vi "Data_Save_ECO.vi"(9 "Data":T1) -> (2 "Eco":string[](array[string]))   [LabVIEW 2017]
uses:
  Ctrls/Data.ctl
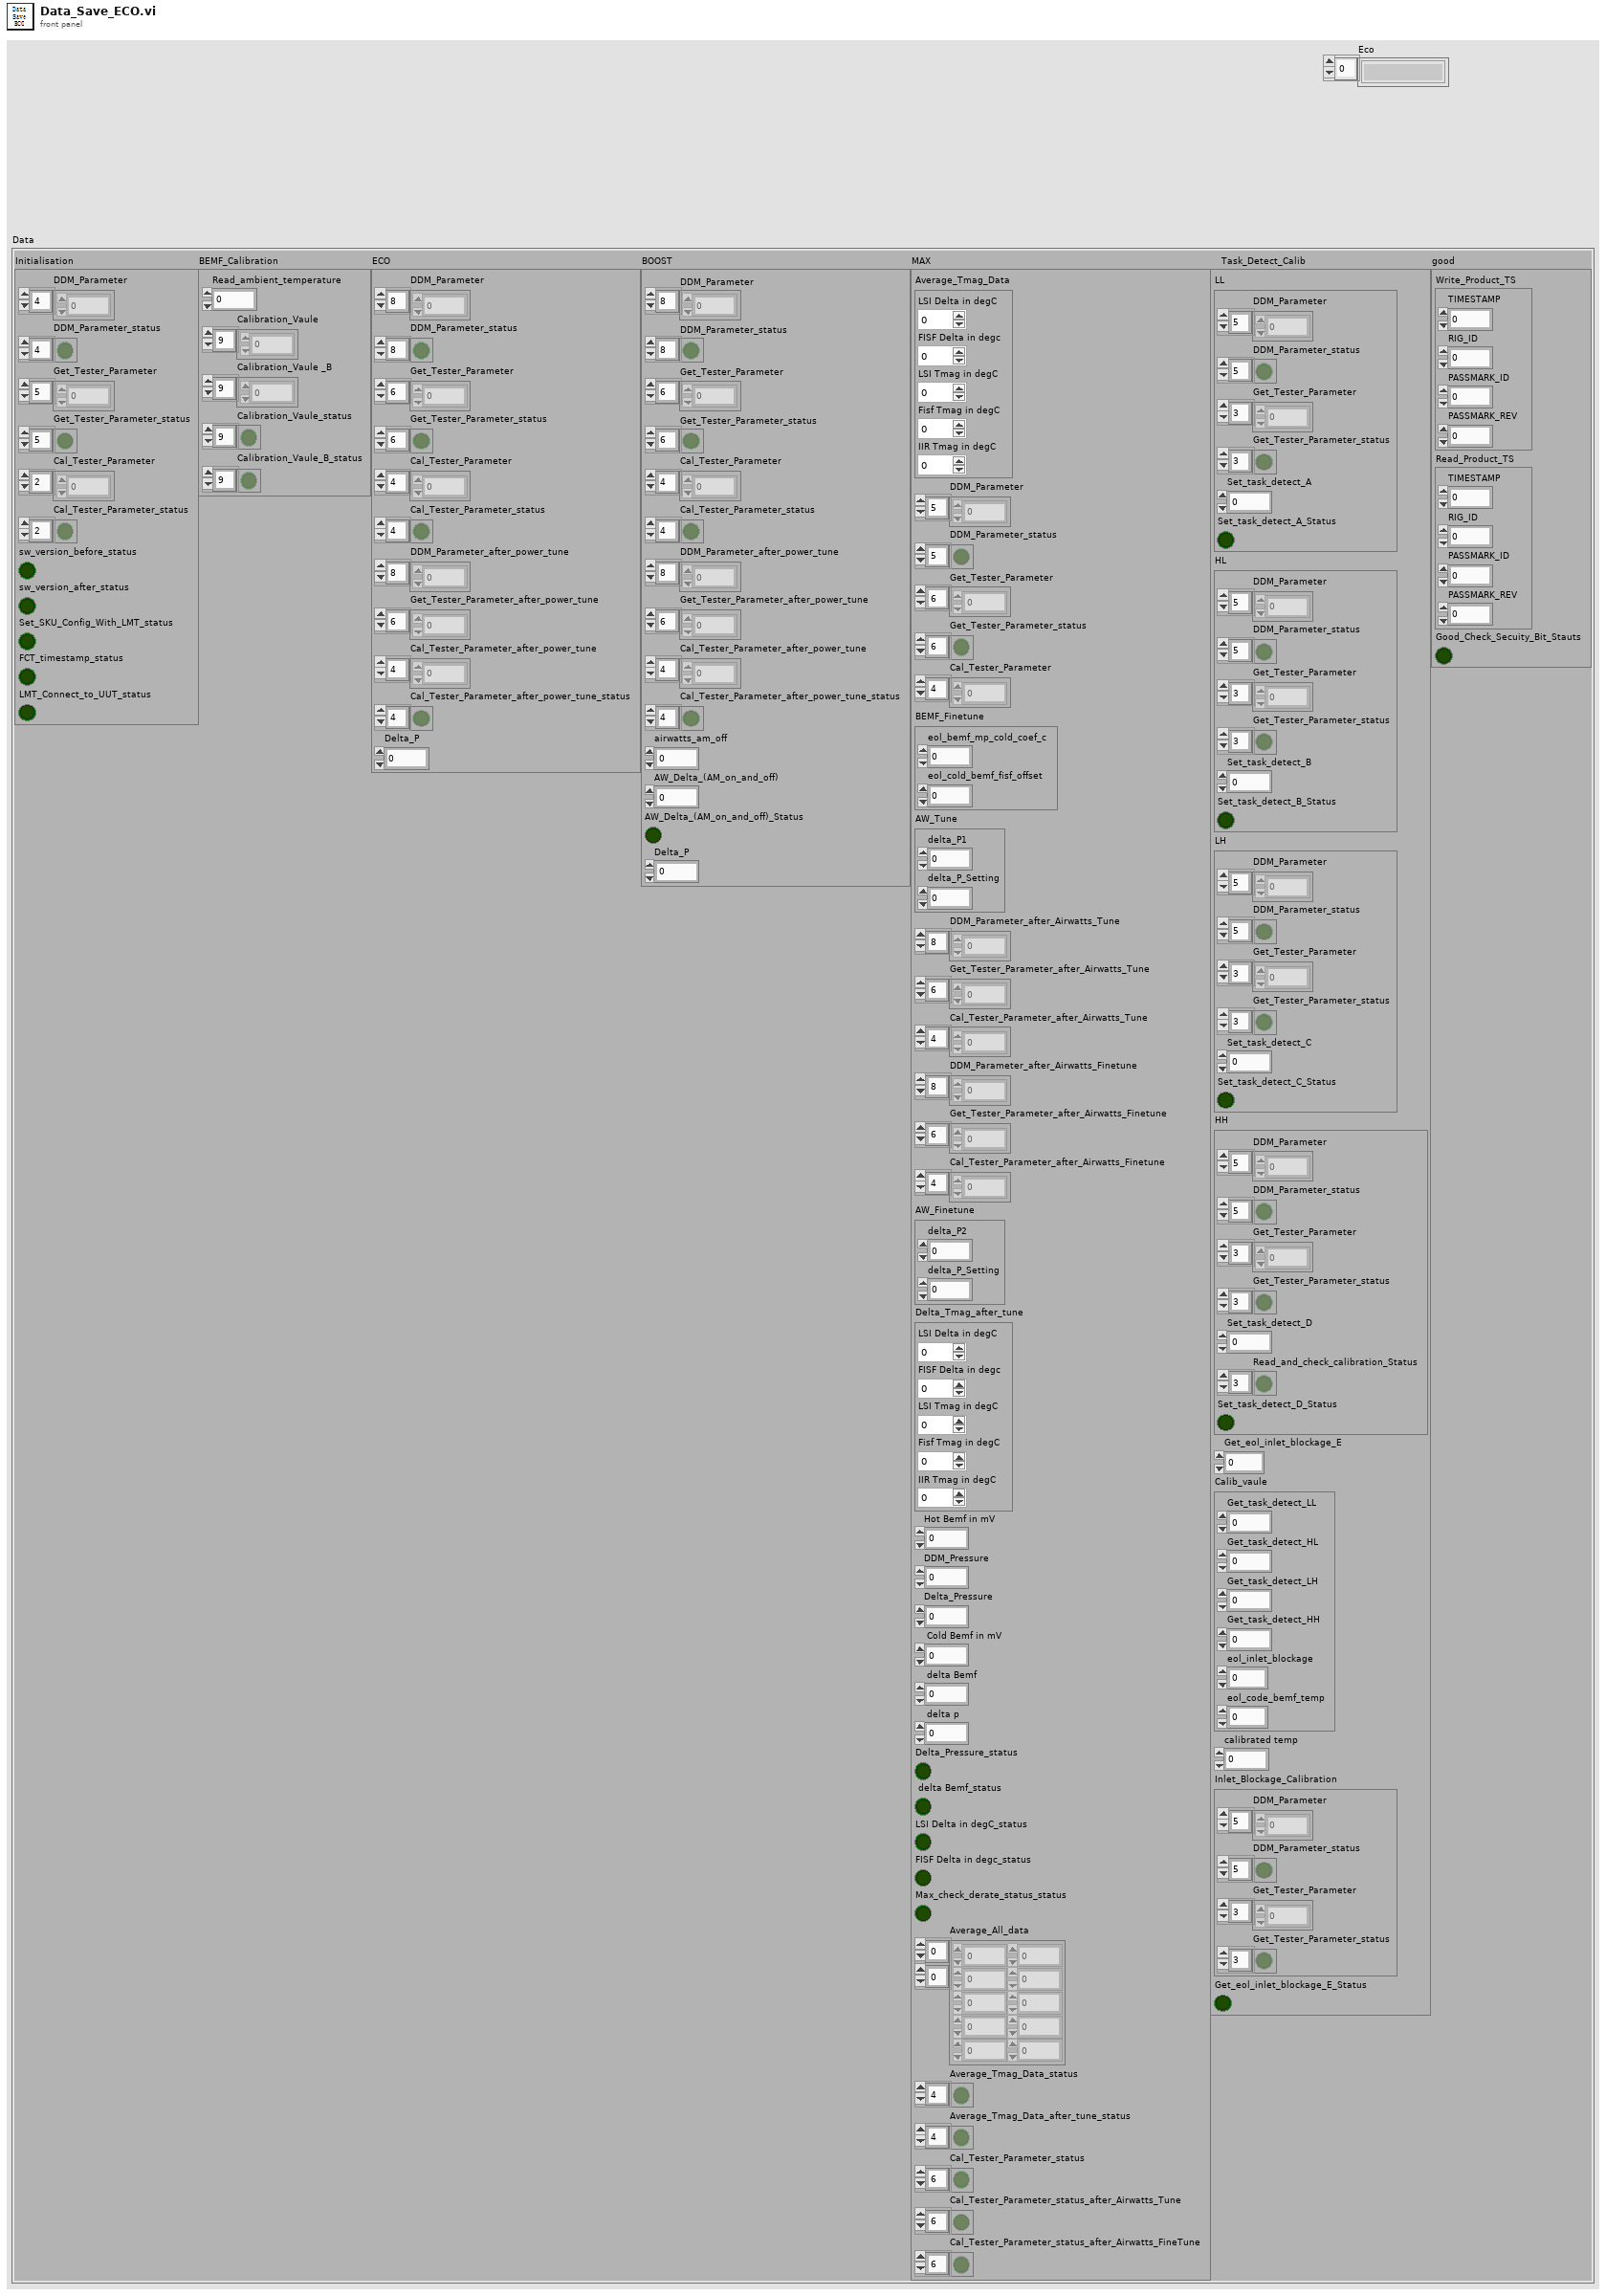
[diagram p1: front panel]
types:
  T1 = typedef "Data.ctl" = cluster{"Initialisation":cluster{"DDM_Parameter":dbl[], "DDM_Parameter_status":bool[], "Get_Tester_Parameter":dbl[], "Get_Tester_Parameter_status":bool[], "Cal_Tester_Parameter":dbl[], "Cal_Tester_Parameter_status":bool[], "sw_version_before_status":bool, "sw_version_after_status":bool, "Set_SKU_Config_With_LMT_status":bool, "FCT_timestamp_status":bool, "LMT_Connect_to_UUT_status":bool}, "BEMF_Calibration":cluster{"Read_ambient_temperature":dbl, "Calibration_Vaule":dbl[], "Calibration_Vaule _B":dbl[], "Calibration_Vaule_status":bool[], "Calibration_Vaule_B_status":bool[]}, "ECO":cluster{"DDM_Parameter":dbl[], "DDM_Parameter_status":bool[], "Get_Tester_Parameter":dbl[], "Get_Tester_Parameter_status":bool[], "Cal_Tester_Parameter":dbl[], "Cal_Tester_Parameter_status":bool[], "DDM_Parameter_after_power_tune":dbl[], "Get_Tester_Parameter_after_power_tune":dbl[], "Cal_Tester_Parameter_after_power_tune":dbl[], "Cal_Tester_Parameter_after_power_tune_status":bool[], "Delta_P":dbl}, "BOOST":cluster{"DDM_Parameter":dbl[], "DDM_Parameter_status":bool[], "Get_Tester_Parameter":dbl[], "Get_Tester_Parameter_status":bool[], "Cal_Tester_Parameter":dbl[], "Cal_Tester_Parameter_status":bool[], "DDM_Parameter_after_power_tune":dbl[], "Get_Tester_Parameter_after_power_tune":dbl[], "Cal_Tester_Parameter_after_power_tune":dbl[], "Cal_Tester_Parameter_after_power_tune_status":bool[], "airwatts_am_off":dbl, "AW_Delta_(AM_on_and_off)":dbl, "AW_Delta_(AM_on_and_off)_Status":bool, "Delta_P":dbl}, "MAX":cluster{"Average_Tmag_Data":cluster{"LSI Delta in degC":dbl, "FISF Delta in degc":dbl, "LSI Tmag in degC":dbl, "Fisf Tmag in degC":dbl, "IIR Tmag in degC":dbl}, "DDM_Parameter":dbl[], "DDM_Parameter_status":bool[], "Get_Tester_Parameter":dbl[], "Get_Tester_Parameter_status":bool[], "Cal_Tester_Parameter":dbl[], "BEMF_Finetune":cluster{"eol_bemf_mp_cold_coef_c":dbl, "eol_cold_bemf_fisf_offset":dbl}, "AW_Tune":cluster{"delta_P1":dbl, "delta_P_Setting":dbl}, "DDM_Parameter_after_Airwatts_Tune":dbl[], "Get_Tester_Parameter_after_Airwatts_Tune":dbl[], "Cal_Tester_Parameter_after_Airwatts_Tune":dbl[], "DDM_Parameter_after_Airwatts_Finetune":dbl[], "Get_Tester_Parameter_after_Airwatts_Finetune":dbl[], "Cal_Tester_Parameter_after_Airwatts_Finetune":dbl[], "AW_Finetune":cluster{"delta_P2":dbl, "delta_P_Setting":dbl}, "Delta_Tmag_after_tune":cluster{"LSI Delta in degC":dbl, "FISF Delta in degc":dbl, "LSI Tmag in degC":dbl, "Fisf Tmag in degC":dbl, "IIR Tmag in degC":dbl}, "Hot Bemf in mV":dbl, "DDM_Pressure":dbl, "Delta_Pressure":dbl, " Cold Bemf in mV":dbl, " delta Bemf":dbl, " delta p":dbl, "Delta_Pressure_status":bool, " delta Bemf_status":bool, "LSI Delta in degC_status":bool, "FISF Delta in degc_status":bool, "Max_check_derate_status_status":bool, "Average_All_data":dbl[][], "Average_Tmag_Data_status":bool[], "Average_Tmag_Data_after_tune_status":bool[], "Cal_Tester_Parameter_status":bool[], "Cal_Tester_Parameter_status_after_Airwatts_Tune":bool[], "Cal_Tester_Parameter_status_after_Airwatts_FineTune":bool[]}, "Task_Detect_Calib":cluster{"LL":cluster{"DDM_Parameter":dbl[], "DDM_Parameter_status":bool[], "Get_Tester_Parameter":dbl[], "Get_Tester_Parameter_status":bool[], "Set_task_detect_A":dbl, "Set_task_detect_A_Status":bool}, "HL":cluster{"DDM_Parameter":dbl[], "DDM_Parameter_status":bool[], "Get_Tester_Parameter":dbl[], "Get_Tester_Parameter_status":bool[], "Set_task_detect_B":dbl, "Set_task_detect_B_Status":bool}, "LH":cluster{"DDM_Parameter":dbl[], "DDM_Parameter_status":bool[], "Get_Tester_Parameter":dbl[], "Get_Tester_Parameter_status":bool[], "Set_task_detect_C":dbl, "Set_task_detect_C_Status":bool}, "HH":cluster{"DDM_Parameter":dbl[], "DDM_Parameter_status":bool[], "Get_Tester_Parameter":dbl[], "Get_Tester_Parameter_status":bool[], "Set_task_detect_D":dbl, "Read_and_check_calibration_Status":bool[], "Set_task_detect_D_Status":bool}, "Get_eol_inlet_blockage_E":dbl, "Calib_vaule":cluster{"Get_task_detect_LL":dbl, "Get_task_detect_HL":dbl, "Get_task_detect_LH":dbl, "Get_task_detect_HH":dbl, "eol_inlet_blockage":dbl, "eol_code_bemf_temp":dbl}, "calibrated temp":dbl, "Inlet_Blockage_Calibration":cluster{"DDM_Parameter":dbl[], "DDM_Parameter_status":bool[], "Get_Tester_Parameter":dbl[], "Get_Tester_Parameter_status":bool[]}, "Get_eol_inlet_blockage_E_Status":bool}, "good":cluster{"Write_Product_TS":cluster{"TIMESTAMP":i64, "RIG_ID":i64, "PASSMARK_ID":i64, "PASSMARK_REV":i64}, "Read_Product_TS":cluster{"TIMESTAMP":i64, "RIG_ID":i64, "PASSMARK_ID":i64, "PASSMARK_REV":i64}, "Good_Check_Secuity_Bit_Stauts":bool}}
  T2 = typedef "HD Config.ctl" = cluster{" PC":cluster{"PC Address":u8[], "PC Port":i32}, "FCO":cluster{"COM":refnum<visa-resource-name>, "Baudrate":u32}, "DC Power ":cluster{"COM":refnum<visa-resource-name>, "Baudrate":u32}, "PW3336":cluster{"COM":refnum<visa-resource-name>, "Baudrate":u32}, "Lefoo":cluster{"COM":refnum<visa-resource-name>, "Baudrate":u32}, "AI Model":cluster{"COM":refnum<visa-resource-name>, "Baudrate":u32}, "DIPC":cluster{"COM":refnum<visa-resource-name>}, "Daemon":cluster{"IP Address":string, "Port":u16, "Retry":u16}, "Motor":cluster{"COM":refnum<visa-resource-name>, "Baudrate":u32}, "G1":bool, "Fail_resume_mode":bool, "Skip DDM Speed&Pressure Passmark":bool}
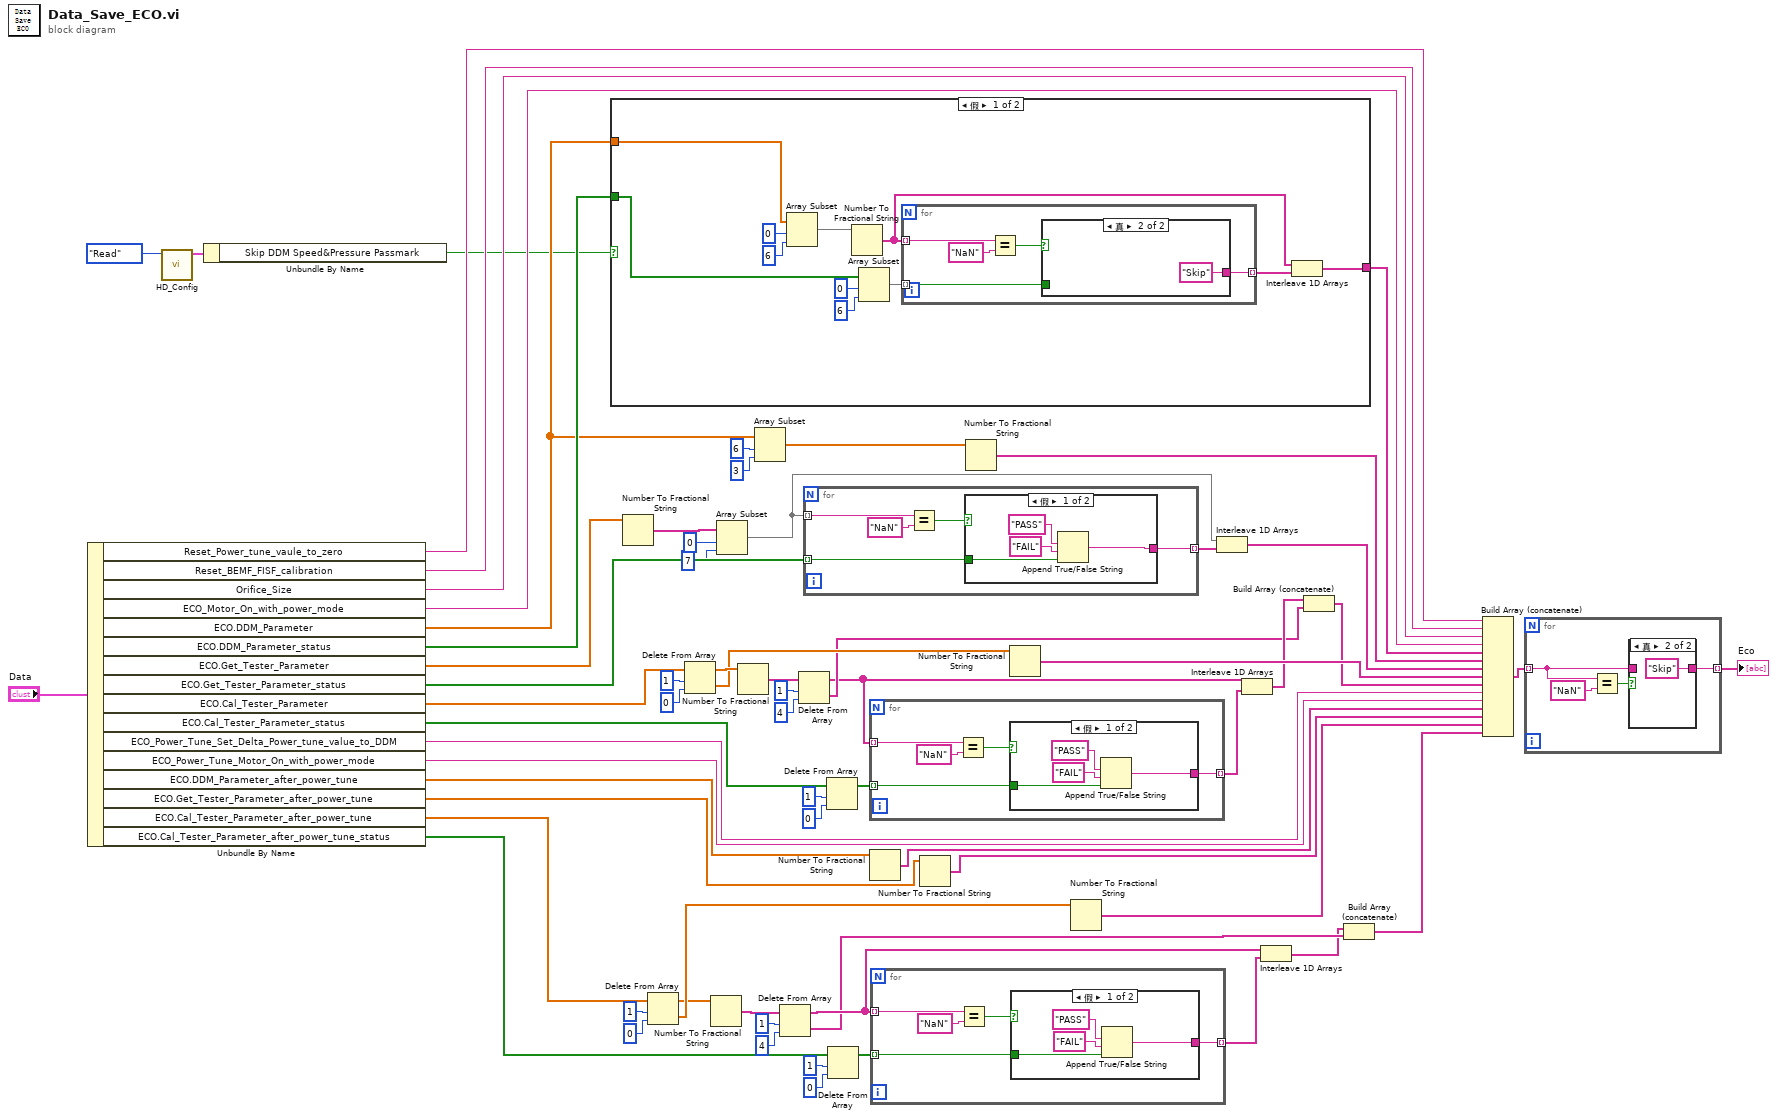
[diagram p0: block diagram]
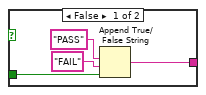
[diagram p2: hidden frame]
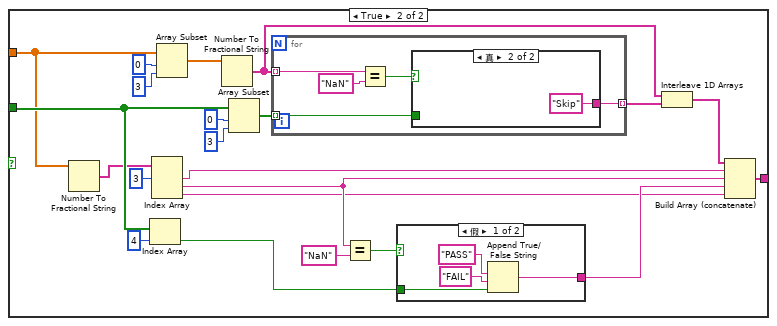
[diagram p3: hidden frame]
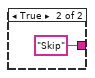
[diagram p4: hidden frame]
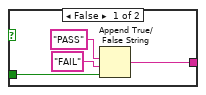
[diagram p5: hidden frame]
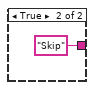
[diagram p7: hidden frame]
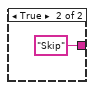
[diagram p8: hidden frame]
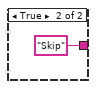
[diagram p9: hidden frame]
diagram:
  n1 = Unbundle By Name("Data") -> ("Reset_Power_tune_vaule_to_zero"=w28:string, "Reset_BEMF_FISF_calibration"=w29:string, "Orifice_Size"=w27:string, "ECO_Motor_On_with_power_mode"=w45:string, "ECO.DDM_Parameter"=w25:dbl[], "ECO.DDM_Parameter_status"=w26:bool[], "ECO.Get_Tester_Parameter"=w20:dbl[], "ECO.Get_Tester_Parameter_status"=w42:bool[], "ECO.Cal_Tester_Parameter"=w61:dbl[], "ECO.Cal_Tester_Parameter_status"=w56:bool[], "ECO_Power_Tune_Set_Delta_Power_tune_value_to_DDM"=w44:string, "ECO_Power_Tune_Motor_On_with_power_mode"=w43:string, "ECO.DDM_Parameter_after_power_tune"=w66:dbl[], "ECO.Get_Tester_Parameter_after_power_tune"=w67:dbl[], "ECO.Cal_Tester_Parameter_after_power_tune"=w47:dbl[], "ECO.Cal_Tester_Parameter_after_power_tune_status"=w46:bool[])
  n2 = call "HD_Config.vi"("Step"=enum16{"Initial", "Write", "Read"}."Read") -> ("HD Config out"=w22:T2)  [unwired: 9 in, 1 out]
  n3 = Unbundle By Name(w22) -> ("Skip DDM Speed&Pressure Passmark"=w21:bool)
  n4 = case shown="假" w21 {
    tunnel: w26 -> [w69 w100]
    tunnel: w25 -> [w70 w97]
    tunnel: [w68 w89] -> w24
    frame False {
      n5 = Array Subset(array=w70, index=0 ("索引"), length=6 ("长度")) -> (w76:dbl[])
      n6 = Number To Fractional String(number=w76) -> (F-format string=w75:string[])  [unwired: 3 in]
      n7 = Array Subset(array=w69, index=0 ("索引"), length=6 ("长度")) -> (w77:bool[])
      n8 = for {
        tunnel: w77 -> [w83] mode=indexing
        tunnel: [w82] -> w78 mode=indexing
        tunnel: w75 -> [w80] mode=indexing
        n9 = Equal?(x=w80, y="NaN" ("x")) -> (x = y?=w79:bool)
        n10 = case shown="真" w79 {
          tunnel: w83 -> [w87 _]
          tunnel: [w85 "Skip" ("x")] -> w82
          frame False {
            n11 = Append True/False String(1:w87, 2:"FAIL" ("字符串(\"\")"), 3:"PASS" ("真字符串")) -> (0:w85:string)  [unwired: 1 in]
          }
          frame True {
          }
        }
      }
      n12 = Interleave 1D Arrays(w75, w78) -> (w68:string[])
    }
    frame True {
      n13 = Number To Fractional String(number=w97) -> (F-format string=w96:string[])  [unwired: 3 in]
      n14 = Index Array(array=w100, index=4 ("索引")) -> (element=w95:bool)
      n15 = Index Array(array=w96, index #1=3 ("索引")) -> (element #1=w94:string, element #2=w92:string, element #3=w91:string)  [unwired: 2 in]
      n16 = Array Subset(array=w97, index=0 ("索引"), length=3 ("长度")) -> (w108:dbl[])
      n17 = Number To Fractional String(number=w108) -> (F-format string=w103:string[])  [unwired: 3 in]
      n18 = Array Subset(array=w100, index=0 ("索引"), length=3 ("长度")) -> (w109:bool[])
      n19 = for {
        tunnel: w109 -> [w120] mode=indexing
        tunnel: [w119] -> w110 mode=indexing
        tunnel: w103 -> [w117] mode=indexing
        n20 = Equal?(x=w117, y="NaN" ("x")) -> (x = y?=w116:bool)
        n21 = case shown="真" w116 {
          tunnel: w120 -> [w124 _]
          tunnel: [w122 "Skip" ("x")] -> w119
          frame False {
            n22 = Append True/False String(1:w124, 2:"FAIL" ("字符串(\"\")"), 3:"PASS" ("真字符串")) -> (0:w122:string)  [unwired: 1 in]
          }
          frame True {
          }
        }
      }
      n23 = Equal?(x=w92, y="NaN" ("x")) -> (x = y?=w99:bool)
      n24 = case shown="假" w99 {
        tunnel: w95 -> [w114 _]
        tunnel: [w112 "Skip" ("x")] -> w93
        frame False {
          n25 = Append True/False String(1:w114, 2:"FAIL" ("字符串(\"\")"), 3:"PASS" ("真字符串")) -> (0:w112:string)  [unwired: 1 in]
        }
        frame True {
        }
      }
      n26 = Interleave 1D Arrays(w103, w110) -> (w90:string[])
      n27 = Build Array (concatenate)(w90, w94, w92, w93, w91) -> (w89:string[])
    }
  }
  n28 = Number To Fractional String(number=w20) -> (F-format string=w16:string[])  [unwired: 3 in]
  n29 = Delete From Array(array=w47, length=1 ("长度"), index=0 ("索引")) -> (deleted portion=w51:dbl[], array with subset deleted=w50:dbl[])
  n30 = Delete From Array(array=w61, length=1 ("长度"), index=0 ("索引")) -> (deleted portion=w57:dbl[], array with subset deleted=w58:dbl[])
  n31 = Number To Fractional String(number=w50) -> (F-format string=w5:string[])  [unwired: 3 in]
  n32 = Array Subset(array=w16, index=0 ("索引"), length=7 ("长度")) -> (w19:string[])
  n33 = Number To Fractional String(number=w58) -> (F-format string=w10:string[])  [unwired: 3 in]
  n34 = Array Subset(array=w25, index=6 ("索引"), length=3 ("长度")) -> (w65:dbl[])
  n35 = Delete From Array(array=w5, length=1 ("长度"), index=4 ("索引")) -> (deleted portion=w3:string[], array with subset deleted=w4:string[])
  n36 = Delete From Array(array=w10, length=1 ("长度"), index=4 ("索引")) -> (deleted portion=w9:string[], array with subset deleted=w8:string[])
  n37 = for {
    tunnel: w42 -> [w130] mode=indexing
    tunnel: [w129] -> w41 mode=indexing
    tunnel: w19 -> [w127] mode=indexing
    n38 = Equal?(x=w127, y="NaN" ("x")) -> (x = y?=w126:bool)
    n39 = case shown="假" w126 {
      tunnel: w130 -> [w134 _]
      tunnel: [w132 "Skip" ("x")] -> w129
      frame False {
        n40 = Append True/False String(1:w134, 2:"FAIL" ("字符串(\"\")"), 3:"PASS" ("真字符串")) -> (0:w132:string)  [unwired: 1 in]
      }
      frame True {
      }
    }
  }
  n41 = Delete From Array(array=w56, length=1 ("长度"), index=0 ("索引")) -> (array with subset deleted=w40:bool[])  [unwired: 1 out]
  n42 = Delete From Array(array=w46, length=1 ("长度"), index=0 ("索引")) -> (array with subset deleted=w38:bool[])  [unwired: 1 out]
  n43 = for {
    tunnel: w40 -> [w140] mode=indexing
    tunnel: [w139] -> w39 mode=indexing
    tunnel: w8 -> [w137] mode=indexing
    n44 = Equal?(x=w137, y="NaN" ("x")) -> (x = y?=w136:bool)
    n45 = case shown="假" w136 {
      tunnel: w140 -> [w144 _]
      tunnel: [w142 "Skip" ("x")] -> w139
      frame False {
        n46 = Append True/False String(1:w144, 2:"FAIL" ("字符串(\"\")"), 3:"PASS" ("真字符串")) -> (0:w142:string)  [unwired: 1 in]
      }
      frame True {
      }
    }
  }
  n47 = Number To Fractional String(number=w66) -> (F-format string=w34:string[])  [unwired: 3 in]
  n48 = for {
    tunnel: w38 -> [w150] mode=indexing
    tunnel: [w149] -> w37 mode=indexing
    tunnel: w4 -> [w147] mode=indexing
    n49 = Equal?(x=w147, y="NaN" ("x")) -> (x = y?=w146:bool)
    n50 = case shown="假" w146 {
      tunnel: w150 -> [w154 _]
      tunnel: [w152 "Skip" ("x")] -> w149
      frame False {
        n51 = Append True/False String(1:w154, 2:"FAIL" ("字符串(\"\")"), 3:"PASS" ("真字符串")) -> (0:w152:string)  [unwired: 1 in]
      }
      frame True {
      }
    }
  }
  n52 = Number To Fractional String(number=w67) -> (F-format string=w33:string[])  [unwired: 3 in]
  n53 = Number To Fractional String(number=w65) -> (F-format string=w35:string[])  [unwired: 3 in]
  n54 = Number To Fractional String(number=w57) -> (F-format string=w36:string[])  [unwired: 3 in]
  n55 = Number To Fractional String(number=w51) -> (F-format string=w32:string[])  [unwired: 3 in]
  n56 = Interleave 1D Arrays(w19, w41) -> (w15:string[])
  n57 = Interleave 1D Arrays(w8, w39) -> (w14:string[])
  n58 = Interleave 1D Arrays(w4, w37) -> (w2:string[])
  n59 = Build Array (concatenate)(w14, w9) -> (w13:string[])
  n60 = Build Array (concatenate)(w2, w3) -> (w1:string[])
  n61 = Build Array (concatenate)(w28, w29, w27, w45, w24, w35, w15, w36, w13, w44, w43, w34, w33, w32, w1) -> (w31:string[])
  n62 = for {
    tunnel: [w159] -> w30 mode=indexing
    tunnel: w31 -> [w156] mode=indexing
    n63 = Equal?(x=w156, y="NaN" ("x")) -> (x = y?=w157:bool)
    n64 = case shown="真" w157 {
      tunnel: [w160 "Skip" ("x")] -> w159
      tunnel: w156 -> [w160 _]
      frame False {
      }
      frame True {
      }
    }
  }
  "Eco" <- w30
